vi "InitialConstI6221.vi"(2 "error in (no error)":errorcluster, 3 "Amplitude In (A)":dbl, 4 "VISA Refnum in":refnum<visa-resource-name>) -> (0 "error out":errorcluster, 1 "VISA Refnum out":refnum<visa-resource-name>)   [LabVIEW 2012]
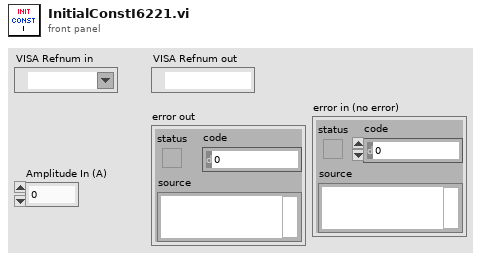
[diagram p1: front panel]
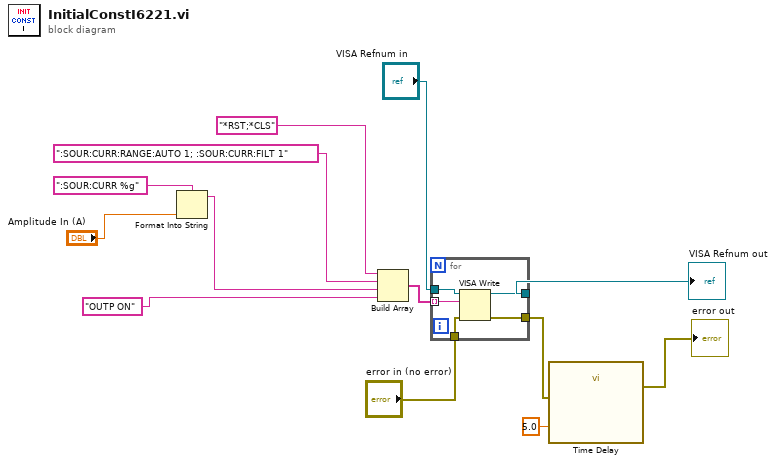
[diagram p0: block diagram]
diagram:
  n1 = Format Into String(format string=":SOUR:CURR %g", "Amplitude In (A)") -> (resulting string=w4:string)  [unwired: 2 in, 1 out]
  n2 = Build Array("*RST;*CLS" ("write buffer"), ":SOUR:CURR:RANGE:AUTO 1; :SOUR:CURR:FILT 1" ("write buffer"), w4, "OUTP ON" ("format string")) -> (w11:string[])
  n3 = for {
    tunnel: w11 -> [w18] mode=indexing
    tunnel: "VISA Refnum in" -> [w17]
    tunnel: [w16] -> w13
    tunnel: [w15] -> w10
    tunnel: "error in (no error)" -> [w14]
    n4 = VISA Write(VISA resource name=w17, write buffer=w18, error in (no error)=w14) -> (VISA resource name out=w16:refnum<visa-resource-name>, error out=w15:errorcluster)  [unwired: 1 out]
  }
  "VISA Refnum out" <- w13
  n5 = call "Time Delay"("error in (no error)"=w10, "Delay Time (s)"=5.0) -> ("error out"=→"error out":errorcluster)  [unwired: 9 in]
